vi "_MIIPS.vi"() -> ()   [LabVIEW 2022 SP3]
uses:
  <vilib>/Analysis/2dsp.llb/Integral Method.ctl
  Global 1.vi
  <vilib>/Analysis/NI_AALPro.lvlib
panel:
  out "SLM":bool
  out "Current iteration":i32
  out "cursors":T1(array[cluster])
  in  "wl start":dbl=765.0
  in  "wl end":dbl=825.0
  out "SLM file status":bool
  out "SLM mask file":path
  out "Raw phase status":bool
  out "File location":path=path "MIIPS_phase.txt"
  in  "Phase folder":path=path "C:/Alexander/LabView programs/SLM/Calibration Data"
  in  "Stop":bool
  in  "SHG spectrometer file":path=path "C:/Data/Data/spec1.xls"
  in  "Master Mask Calibration":path=path "C:/Alexander/LabView programs/SLM/Calibration Data/master scanning.txt"
  in  "Slave Mask Calibration":path=path "C:/Alexander/LabView programs/SLM/Calibration Data/slave scanning.txt"
  in  "SLM COM Port":refnum<visa-resource-name>="COM9"
  out "second derivative":string
  out "reference function":string
  in  "Gamma (fs)":ext=59.0
  in  "Alpha (rad)":dbl=6.0
  in  "Termination":cluster{"Threshold":dbl, "Max iterations":i32}={"Threshold"=0.0, "Max iterations"=4}
  out "Traces":cluster{"Trace":dbl[][]}[](array[cluster])
  out "Phases":T2(graph)
  in  "Delta increment (rad)":dbl=0.1
  # "Wavelength range (nm)"
  # "–"
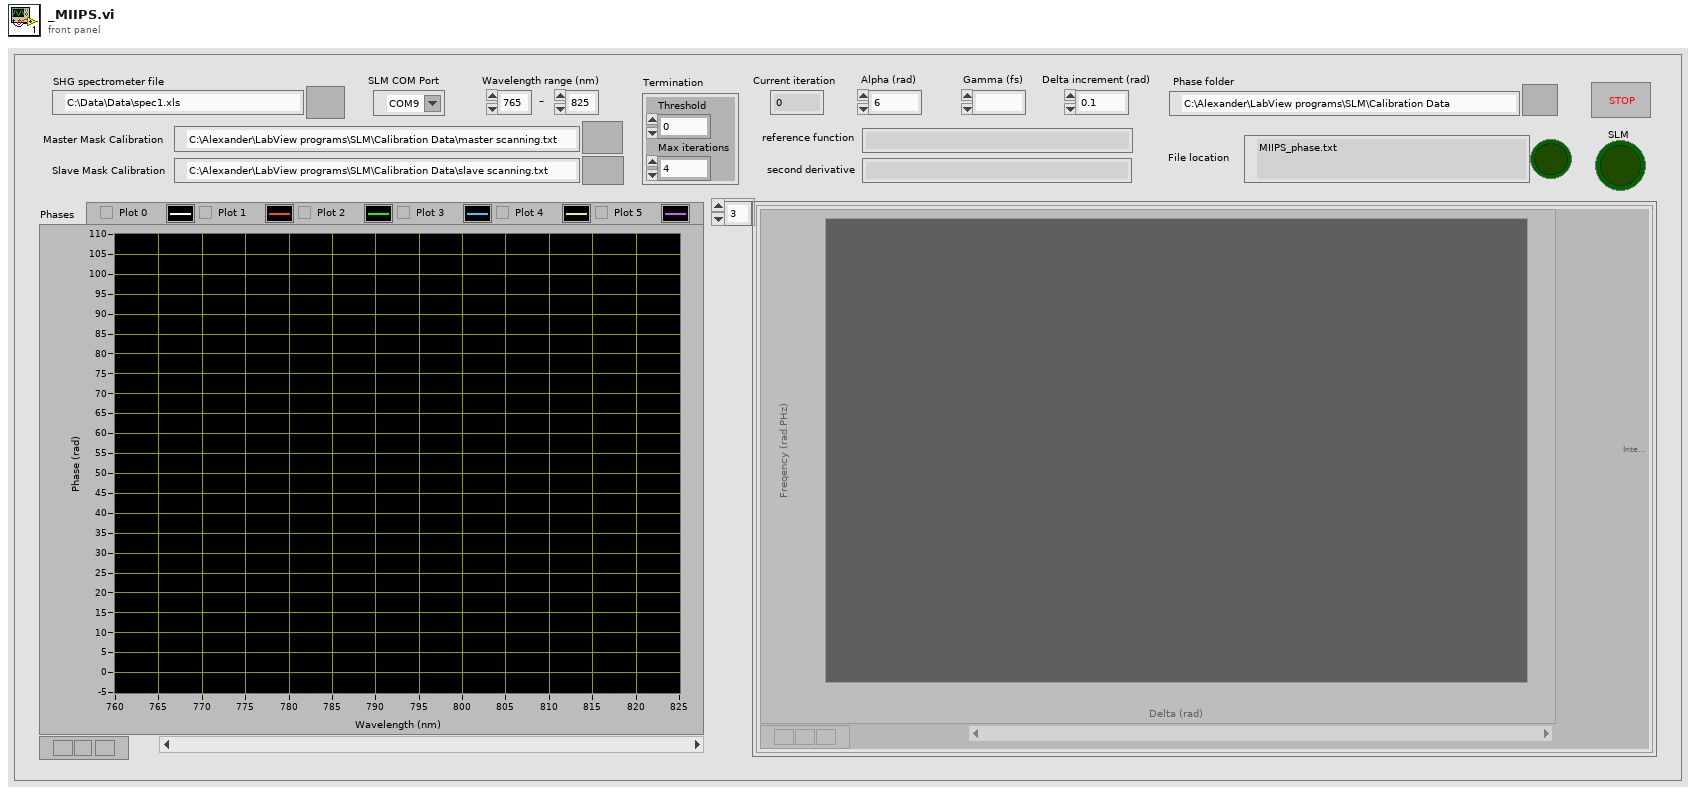
[diagram p1: front panel]
types:
  T1 = cluster{string, i32, i32, i32, bool, bool, i32, i32, i32, cluster{"Numeric":dbl, dbl}, i32, i32, i32[], bool, i32, cluster{dbl, dbl}}[][]
  T2 = cluster{"Integral X":dbl[], "Integral X":dbl[]}[]
  T3 = cluster{"Y Values":dbl[][], "Tables":i32[][][], "Variables input decode":i32[], "Variables output decode":i32[]}
  T4 = typedef "NI_AALPro.lvlib/Integral Method.ctl" = i32
  T5 = cluster{"delta inc":dbl, dbl, "freq inc":dbl, dbl}
  T6 = cluster{string, i32, i32, i32, bool, bool, i32, i32, i32, cluster{"Numeric":dbl, dbl}, i32, i32, i32[], bool, i32, cluster{dbl, dbl}}[]
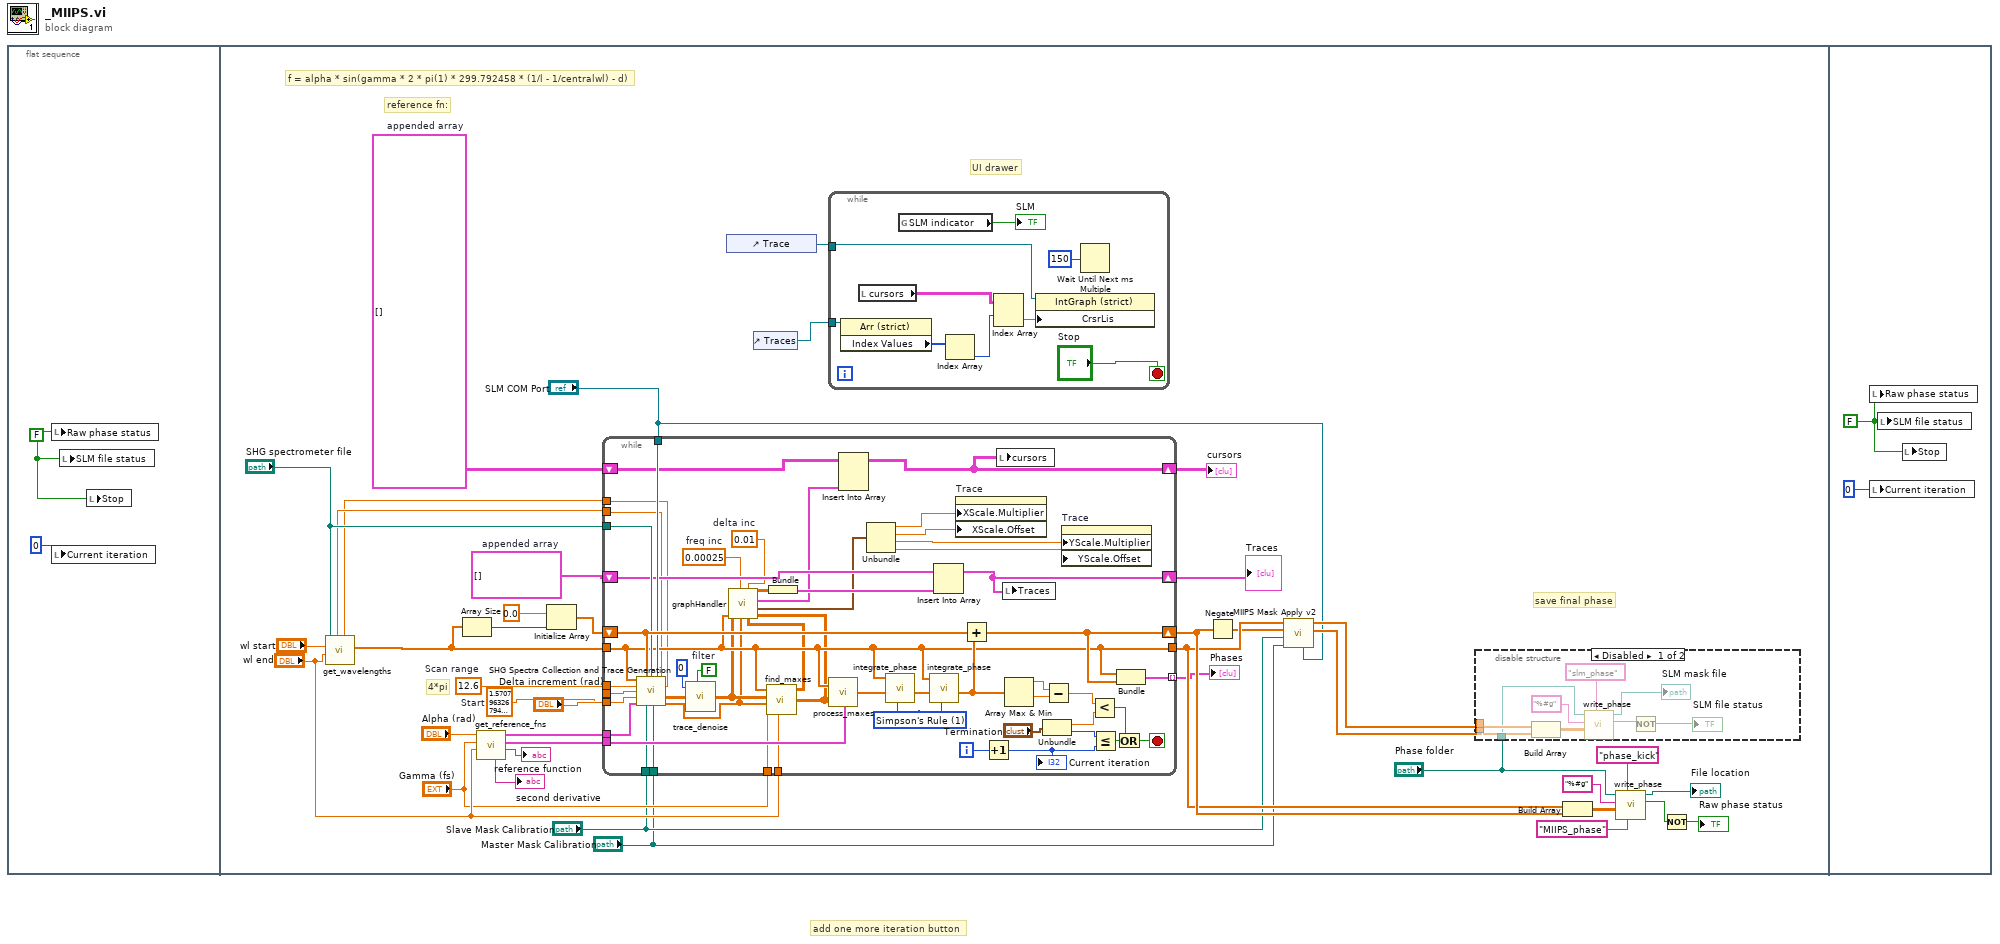
[diagram p0: block diagram]
diagram:
  # "add one more iteration button"
  n1 = flat-sequence {
    frame #0 {
      w1 = FALSE
      n2 = local write "Raw phase status"(w1) -> ()
      n3 = local write "Current iteration"(0) -> ()
      n4 = local write "SLM file status"(w1) -> ()
      n5 = local write "Stop"(w1) -> ()
    }
    frame #1 {
      w7 = T1 []  # appended array
      w9 = cluster{"output trace (r=d, c=freq)":dbl[][]}[] []  # appended array
      w18 = 1.5707963267948966  # Start
      w33 = 12.6  # Scan range
      # "UI drawer"
      # "save final phase"
      # "4*pi"
      # "reference fn:"
      # "f = alpha * sin(gamma * 2 * pi(1) * 299.792458 * (1/l - 1/centralwl) - d)"
      n6 = call "get_wavelengths.vi"("wl end"="wl end", "wl start"="wl start", "file path (dialog if empty)"="SHG spectrometer file") -> ("Wavelengths"=w42:dbl[], "length"=w40:dbl, "start"=w41:dbl)  [unwired: 6 in]
      n7 = Array Size(array=w42) -> (size(s)=w17:i32)
      n8 = call "get_reference_fns.vi"("Central wavelength (nm)"="wl end", "Gamma"="Gamma (fs)", "Alpha"="Alpha (rad)") -> (1:"reference"=→"reference function":string, 2:"second derivative reference"=w29:T3, 3:"reference"=w30:T3, 4:"second derivative reference"=→"second derivative":string)  [unwired: 5 in]
      n9 = Initialize Array(0.0, w17) -> (w23:dbl[])
      n10 = while {
        tunnel: w33 -> [w114]
        tunnel: "Delta increment (rad)" -> [w113]
        shift-right: [w102] -> w39
        shift-left: w23 -> [w93]
        tunnel: [w103] -> w31 mode=indexing
        tunnel: w30 -> [w101]
        tunnel: w29 -> [w100]
        tunnel: w42 -> [w87]
        tunnel: [w87] -> w38
        tunnel: "Gamma (fs)" -> [w95]
        tunnel: "wl end" -> [w94]
        tunnel: "SLM COM Port" -> [w92]
        tunnel: "Slave Mask Calibration" -> [w91]
        tunnel: "Master Mask Calibration" -> [w90]
        tunnel: w18 -> [w89]
        tunnel: "SHG spectrometer file" -> [w88]
        tunnel: w41 -> [w74]
        tunnel: w40 -> [w73]
        shift-right: [w77] -> w8
        shift-left: w9 -> [w79]
        shift-right: [w65] -> w6
        shift-left: w7 -> [w67]
        i -> [w63]
        stop <- w107 stop-if-true
        w64 = FALSE  # filter
        w76 = 0.00025  # freq inc
        w75 = 0.01  # delta inc
        w96 = T4 1 items=["Trapezoidal Rule", "Simpson's Rule", "Simpson's 3/8 Rule", "Bode Rule"] ("integration method")
        n11 = call "SHG Spectra Collection and Trace Generation.vi"("Wavelengths"=w87, "Net Phase"=w93, "File (SHG Spectra)"=w88, "SLM COM Port"=w92, 4:"Start"=w74, "Scan range"=w114, "Length"=w73, 7:"Start"=w89, "Increment"=w113, "Parsed formula node reference function"=w101, "Slave Mask Calibration"=w91, "Master Mask Calibration"=w90) -> ("Trace (r=wl, c=d)"=w83:dbl[][], "Deltas"=w81:dbl[])  [unwired: 2 in]
        n12 = call "trace_denoise.vi"("filter type"=0, "filter"=w64, "Trace (r=wl, c=d)"=w83) -> ("Denoised trace"=w82:dbl[][])  [unwired: 4 in]
        n13 = call "find_maxes.vi"("Wavelengths"=w87, "Trace (r=wl, c=d)"=w82, "Deltas"=w81, "Gamma"=w95, "WL central"=w94) -> ("Bounds"=w84:dbl[][], "Maxes"=w85:dbl[][])  [unwired: 1 in]
        n14 = call "graphHandler.vi"("Maxes[wl]"=w85, "Bounds[wl]"=w84, "delta inc"=w75, "deltas"=w81, "freq inc"=w76, "wavelengths"=w87, "trace (r=wl, c=d)"=w82) -> ("Scale mult/offset"=w68:T5, "Cursors"=w66:T6, "output trace (r=d, c=freq)"=w86:dbl[][])  [unwired: 2 in]
        n15 = Bundle("output trace (r=d, c=freq)"=w86) -> (w78:cluster{"output trace (r=d, c=freq)":dbl[][]})  [unwired: 1 in]
        n16 = call "process_maxes.vi"("Parsed formula node reference fn 2nd derivative"=w100, "Maxes"=w85, "Wavelengths"=w87) -> ("Phase''"=w99:dbl[])
        n17 = Insert Into Array(array=w67, new element=w66) -> (w65:T1)  [unwired: 2 in]
        n18 = Unbundle(w68) -> ("delta inc"=w69:dbl, w70:dbl, "freq inc"=w71:dbl, w72:dbl)
        n19 = call "integrate_phase.vi"("integration method"=w96, "Integrand (function of wl) (units)"=w99, "Wavelengths (ascending, evenly spaced) (nm)"=w87) -> ("Integral (function of wl) (10^15*units)"=w98:dbl[])  [unwired: 8 in]
        n20 = call "integrate_phase.vi"("integration method"=w96, "Integrand (function of wl) (units)"=w98, "Wavelengths (ascending, evenly spaced) (nm)"=w87) -> ("Integral (function of wl) (10^15*units)"=w97:dbl[])  [unwired: 8 in]
        n21 = Insert Into Array(array=w79, new element=w78) -> (w77:cluster{"output trace (r=d, c=freq)":dbl[][]}[])  [unwired: 1 in]
        n22 = property on="Trace" class="IntGraph (strict)"("XScale.Multiplier"=w69, "XScale.Offset"=w70) -> ()  [unwired: 2 in, 2 out]
        n23 = Add(x=w93, y=w97) -> (x+y=w102:dbl[])
        n24 = Increment(x=w63) -> (x+1=w62:i32)
        "Current iteration" <- w62
        n25 = local write "cursors"(w65) -> ()
        n26 = local write "Traces"(w77) -> ()
        n27 = Array Max & Min(array=w97) -> (max value=w111:dbl, min value=w110:dbl)  [unwired: 2 out]
        n28 = Unbundle("Termination") -> ("Threshold"=w105:dbl, "Max iterations"=w104:i32)
        n29 = Subtract(x=w111, y=w110) -> (x-y=w106:dbl)
        n30 = property on="Trace" class="IntGraph (strict)"("YScale.Multiplier"=w71, "YScale.Offset"=w72) -> ()  [unwired: 2 in, 2 out]
        n31 = Less?(x=w106, y=w105) -> (x < y?=w109:bool)
        n32 = Less Or Equal?(x=w104, y=w62) -> (x <= y?=w108:bool)
        n33 = Or(x=w109, y=w108) -> (x .or. y?=w107:bool)
        n34 = Bundle("Wavelengths"=w87, w102) -> (w103:cluster{"Wavelengths":dbl[], dbl[]})  [unwired: 1 in]
      }
      "Phases" <- w31
      "Traces" <- w8
      "cursors" <- w6
      n35 = control-ref of="Trace"() -> (w16:refnum<vi>)
      n36 = control-ref of="Traces"() -> (w15:refnum<vi>)
      n37 = while {
        tunnel: w15 -> [w61]
        tunnel: w16 -> [w60]
        stop <- "Stop" stop-if-true
        n38 = property on="Property Node" class="Arr (strict)"(reference=w61) -> ("Index Values"=w59:u32[])  [unwired: 1 in, 2 out]
        n39 = local read "cursors"() -> (w54:T1)
        n40 = global read "Global 1.vi" "SLM indicator"() -> (→"SLM":bool)
        n41 = Index Array(array=w59) -> (element=w58:u32)  [unwired: 1 in]
        n42 = Index Array(array=w54, index (row)=w58) -> (element=w57:T6)  [unwired: 1 in]
        n43 = property on="Property Node" class="IntGraph (strict)"(reference=w60, "CrsrLis"=w57) -> ()  [unwired: 1 in, 2 out]
        n44 = Wait Until Next ms Multiple(millisecond multiple=u32 150) -> ()  [unwired: 1 out]
      }
      n45 = Negate(x=w39) -> (-x=w22:dbl[])
      n46 = call "MIIPS Mask Apply v2.vi"("SLM COM Port"="SLM COM Port", "Master Mask Calibration"="Master Mask Calibration", "Slave Mask Calibration"="Slave Mask Calibration", "Phase"=w22, "Wavelength"=w38) -> ("Interpolated phase"=w36:dbl[], "Sampled wavelengths"=w37:dbl[])  [unwired: 4 in, 1 out]
      n47 = disable-structure shown="Disabled" {
        disable-tunnel: w37 -> [w52 _]
        disable-tunnel: w36 -> [w51 _]
        disable-tunnel: "Phase folder" -> [w47 _]
        frame Disabled {
          n48 = Build Array(w52, w51) -> (w49:dbl[][])
          n49 = call "write_phase.vi"("Default filename"="slm_phase", "Array"=w49, "format (%.3f)"="%#g", "Phase folder"=w47) -> ("error?"=w45:bool, "new file path (Not A Path if cancelled)"=→"SLM mask file":path)  [unwired: 5 in, 1 out]
          n50 = Not(x=w45) -> (.not. x?=→"SLM file status":bool)
        }
        frame Enabled {
        }
      }
      n51 = Build Array(w38, w39) -> (w13:dbl[][])
      n52 = call "write_phase.vi"("Filename"="MIIPS_phase", "Default filename"="phase_kick", "Array"=w13, "format (%.3f)"="%#g", "Phase folder"="Phase folder") -> ("error?"=w5:bool, "new file path (Not A Path if cancelled)"=→"File location":path)  [unwired: 4 in, 1 out]
      n53 = Not(x=w5) -> (.not. x?=→"Raw phase status":bool)
    }
    frame #2 {
      w115 = FALSE
      n54 = local write "Raw phase status"(w115) -> ()
      n55 = local write "Current iteration"(0) -> ()
      n56 = local write "SLM file status"(w115) -> ()
      n57 = local write "Stop"(w115) -> ()
    }
  }
